vi "PH_PSDBController.set i Attr and open Services.vi"(0 "i ref in":refnum<vi>, 5 "error in":errorcluster) -> (14 "i ref out":refnum<vi>, 16 "i Attributes":T1={"GUI Refs"={"Data Status"=refnum, "Current Shot ID"=refnum, "active Subsystems"=refnum, "Experiment Description"=refnum, "Shot Comment"=refnum, "Experiment"=refnum, "Shottype"=refnum, "Sequencer SM State"=refnum, "Instances with Errors"=refnum}, "Service ID Shot ID"=-1, "Service ID wanted Subsystem"=-1, "Data Status"=0, "Shotinformation"={"Current Experiment ID"=-1, "Current Shot Type"=-1, "Current Comment"=""}, "Data taking?"=FALSE, "Service ID current Shottype"=-1, "Service ID current Experiment"=-1, "Service ID currentShot Comment"=-1, "Service ID possible Shottypes"=-1, "Service ID possible Experiments"=-1, "possible Experiments"=[], "possible Shottypes"=[], "List"=[], "Subsystems Off?"={"PHELIX_Beamline_fs_YLF_BL_Status"=FALSE, "PHELIX_Beamline_ns_BL_Status"=FALSE, "PHELIX_Beamline_PA_Input_BL_Status"=FALSE, "PHELIX_Beamline_PA_MA_BL_Status"=FALSE, "PHELIX_Beamline_MA_Z6_BL_Status"=FALSE, "PHELIX_Beamline_MA_LB_BL_Status"=FALSE, "PHELIX_Beamline_PA_LL_BL_Status"=FALSE}, "PSDB Credentials"={"PW"="N/A", "ID"="N/A", "DS"="N/A"}} {"List"."Info"."Data Status" items=["no info", "no Data collection", "no problem", "Error getting the ID", "Error writing Data", "Error getting the subsystem", "Error getting the Shot ID", "Error getting the Shot Types", "Error getting the Experiments", "Error verifying wanted Shottype", "Error verifying wanted Experiment"]; "Data Status" items=["no info", "no Data collection", "no problem", "Error getting the ID", "Error writing Data", "Error getting the subsystem", "Error getting the Shot ID", "Error getting the Shot Types", "Error getting the Experiments", "Error verifying wanted Shottype", "Error verifying wanted Experiment"]}, 19 "error out":errorcluster)   [LabVIEW 2014, in "PH_PSDBController.lvlib"]
doc: "In this VI own attributes are set."
uses:
  PH_PSDBController.lvlib
  PH_PSDBController.i attribute.ctl
  PH_Basics/PH_PSDBWriter/PH_PSDBWriter.Data Status.ctl
  CSlibraries-extern/psdb_lv/PSDB_Info.ctl
  PH_Basics/PH_Common/Connection/PH_Connection.PSDB Credentials.ctl
  PH_Devices/PH_Beckhoff_Common/PH_Beckhoff_Common.former PSDB classes.ctl
  PH_Basics/PH_Common/PH_Common.lvlib
  PH_Devices/PH_Beckhoff_Common/PH_Beckhoff_Common.lvlib
  PH_Basics/PH_PSDBWriter/PH_PSDBWriter.lvlib
  CSlibraries-extern/psdb_lv/PSDB.lvlib
  CSlibraries/UtilityLib/UtilityLib.lvlib
  CSlibraries-extern/DimLVEvent/LVDimInterface/LVDimInterface.lvlib
  CS_Core/CSSystem/CSSystemLib/CSSystemLib.lvlib
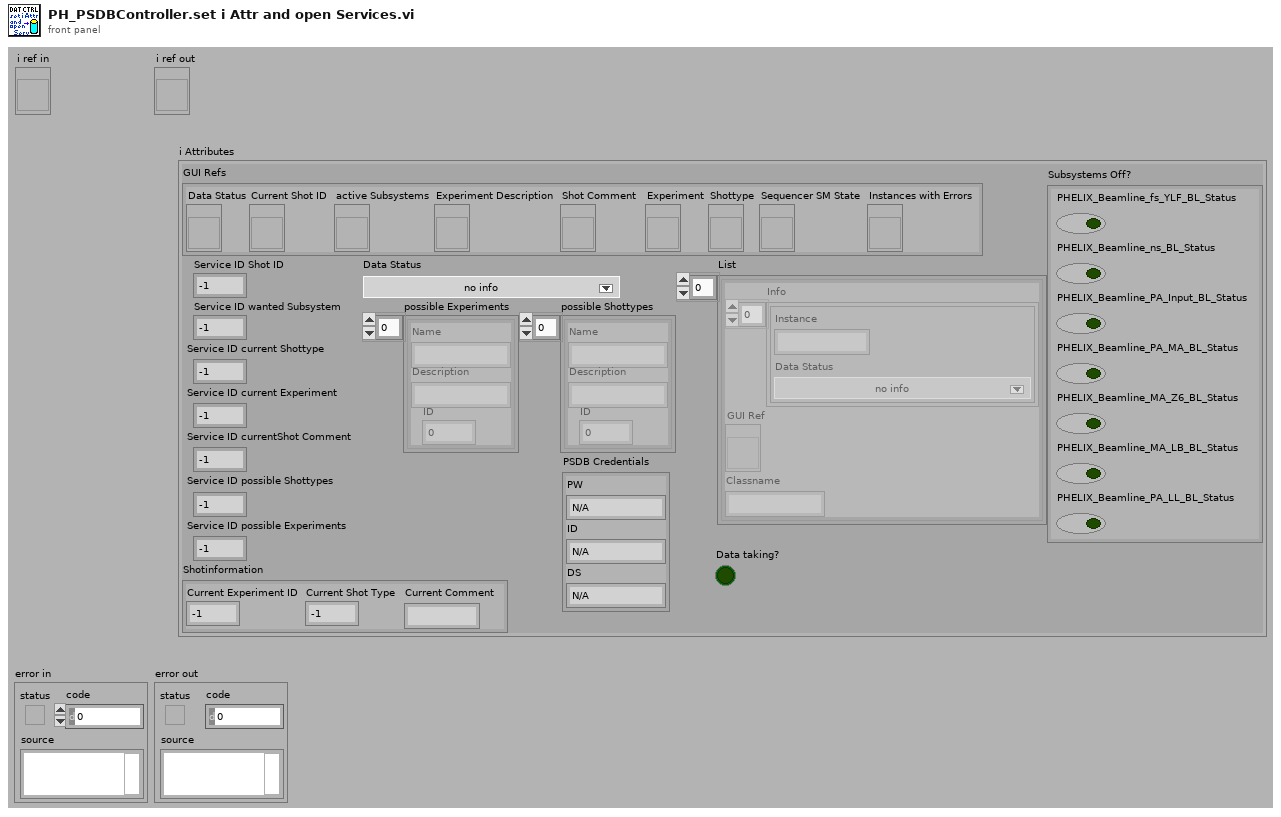
[diagram p1: front panel]
types:
  T1 = typedef "PH_PSDBController.lvlib/PH_PSDBController.i attribute.ctl" = cluster{"GUI Refs":cluster{"Data Status":refnum<vi>, "Current Shot ID":refnum<vi>, "active Subsystems":refnum<vi>, "Experiment Description":refnum<vi>, "Shot Comment":refnum<vi>, "Experiment":refnum<vi>, "Shottype":refnum<vi>, "Sequencer SM State":refnum<vi>, "Instances with Errors":refnum<vi>}, "Service ID Shot ID":i32, "Service ID wanted Subsystem":i32, "Data Status":T2, "Shotinformation":cluster{"Current Experiment ID":i32, "Current Shot Type":i32, "Current Comment":string}, "Data taking?":bool, "Service ID current Shottype":i32, "Service ID current Experiment":i32, "Service ID currentShot Comment":i32, "Service ID possible Shottypes":i32, "Service ID possible Experiments":i32, "possible Experiments":T3[], "possible Shottypes":T3[], "List":cluster{"Info":cluster{"Instance":string, "Data Status":T2}[], "GUI Ref":refnum<vi>, "Classname":string}[], "Subsystems Off?":cluster{"PHELIX_Beamline_fs_YLF_BL_Status":bool, "PHELIX_Beamline_ns_BL_Status":bool, "PHELIX_Beamline_PA_Input_BL_Status":bool, "PHELIX_Beamline_PA_MA_BL_Status":bool, "PHELIX_Beamline_MA_Z6_BL_Status":bool, "PHELIX_Beamline_MA_LB_BL_Status":bool, "PHELIX_Beamline_PA_LL_BL_Status":bool}, "PSDB Credentials":T4}
  T2 = typedef "PH_PSDBWriter.lvlib/PH_PSDBWriter.Data Status.ctl" = i16
  T3 = typedef "PSDB.lvlib/PSDB_Info.ctl" = cluster{"Name":string, "Description":string, "ID":i32}
  T4 = typedef "PH_Common.lvlib/PH_Connection.PSDB Credentials.ctl" = cluster{"PW":string, "ID":string, "DS":string}
  T5 = cluster{"Info":cluster{"Instance":string, "Data Status":T2}[], "GUI Ref":refnum<vi>, "Classname":string}
  T6 = typedef "PH_Beckhoff_Common.lvlib/PH_Beckhoff_Common.former PSDB classes.ctl" = enum16{"PP Conductivity", "PP Mercury", "PA Chiller"}
  T7 = cluster{"Info":cluster{"Instance":string, "Data Status":T2}[], "GUI Ref":refnum<vi>, "Classname":string}[]
  T8 = cluster{"Instancename":string, "Classname":string}
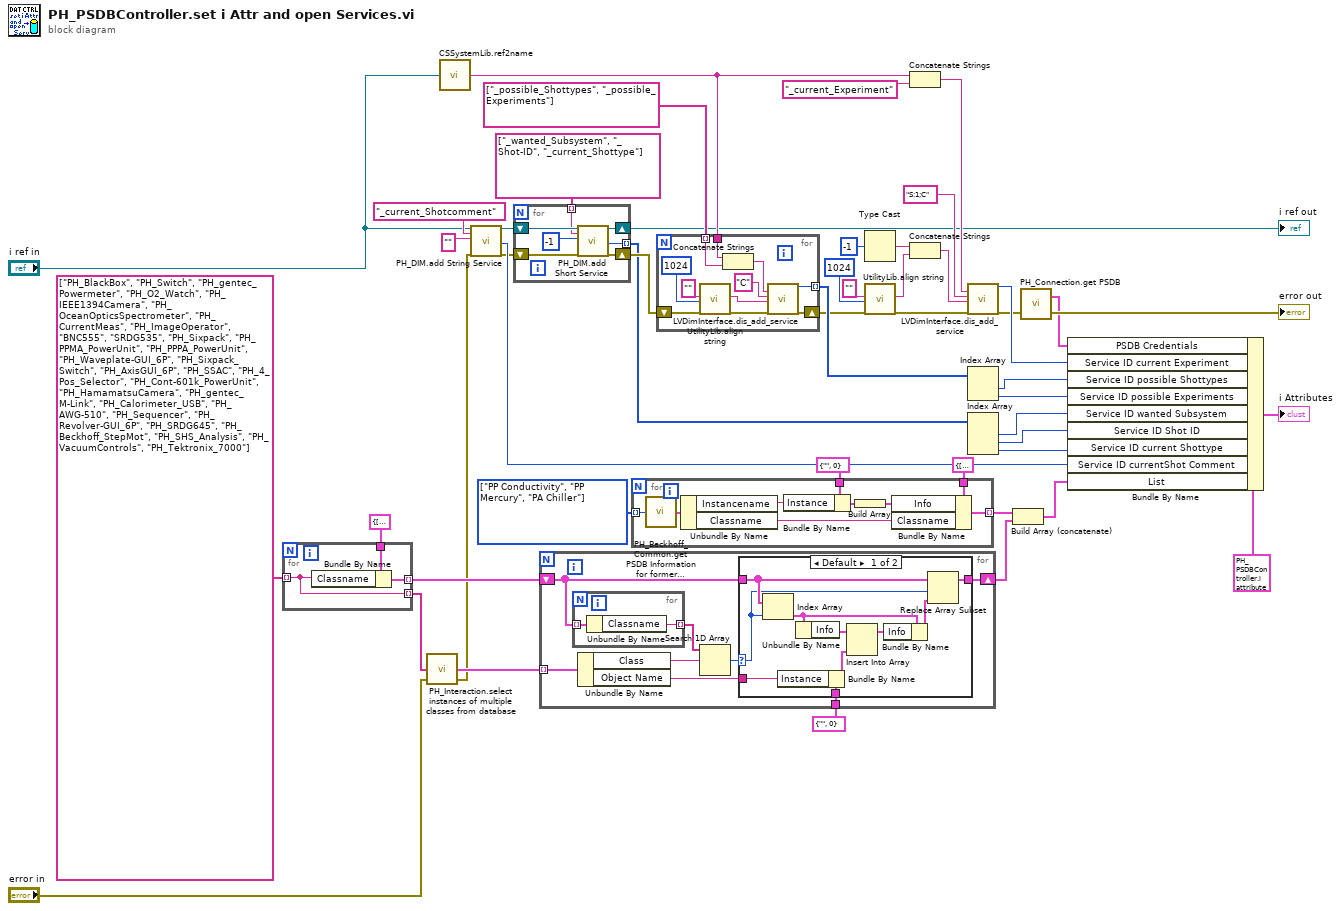
[diagram p0: block diagram]
diagram:
  w45 = T6[] [enum."PP Conductivity", enum."PP Mercury", enum."PA Chiller"] items=["PP Conductivity", "PP Mercury", "PA Chiller"]
  n1 = for {
    tunnel: string[] ["PH_BlackBox", "PH_Switch", "PH_gentec_Powermeter", "PH_O2_Watch", "PH_IEEE1394Camera", "PH_OceanOpticsSpectrometer", "PH_CurrentMeas", "PH_ImageOperator", "BNC555", "SRDG535", "PH_Sixpack", "PH_PPMA_PowerUnit", "PH_PPPA_PowerUnit", "PH_Waveplate-GUI_6P", "PH_Sixpack_Switch", "PH_AxisGUI_6P", "PH_SSAC", "PH_4_Pos_Selector", "PH_Cont-601k_PowerUnit", "PH_HamamatsuCamera", "PH_gentec_M-Link", "PH_Calorimeter_USB", "PH_AWG-510", "PH_Sequencer", "PH_Revolver-GUI_6P", "PH_SRDG645", "PH_Beckhoff_StepMot", "PH_SHS_Analysis", "PH_VacuumControls", "PH_Tektronix_7000"] ("Classes Input") -> [w50] mode=indexing
    tunnel: T5 {"Info"=[], "GUI Ref"=refnum, "Classname"=""} ("Classes") -> [w52]
    tunnel: [w51] -> w46 mode=indexing
    tunnel: [w50] -> w13 mode=indexing
    n2 = Bundle By Name(cluster=w52, "Classname"=w50) -> (w51:T5)
  }
  n3 = call "PH_Interaction.select instances of multiple classes from database.vi"("error in (no error)"="error in", "Classes Input"=w13) -> ("error out"=w8:errorcluster, "Query Result"=w48:cluster{"Object Name":string, "Class":string}[])  [unwired: 2 in]
  n4 = call "CSSystemLib.ref2name.vi"("obj refnum"="i ref in") -> ("name"=w37:string)
  n5 = call "PH_DIM.add String Service.vi"("i ref in"="i ref in", "Service Name"="_current_Shotcomment", "String"="" ("stringIn"), "error in (no error)"=w8) -> ("i ref out"=w19:refnum<vi>, "Service ID"=w21:i32, "error out"=w18:errorcluster)  [unwired: 13 in]
  n6 = for {
    shift-right: [w56] -> w4
    shift-left: w19 -> [w57]
    shift-right: [w58] -> w35
    shift-left: w18 -> [w59]
    tunnel: string[] ["_wanted_Subsystem", "_Shot-ID", "_current_Shottype"] -> [w55] mode=indexing
    tunnel: [w54] -> w15 mode=indexing
    n7 = call "PH_DIM.add Short Service.vi"("i ref in"=w57, "Service Name"=w55, "Number"=i16 -1, "error in (no error)"=w59) -> ("i ref out"=w56:refnum<vi>, "Service ID"=w54:i32, "error out"=w58:errorcluster)  [unwired: 13 in]
  }
  "i ref out" <- w4
  n8 = for {
    tunnel: w48 -> [w67] mode=indexing
    shift-right: [w61] -> w47
    shift-left: w46 -> [w63]
    tunnel: cluster{"Instance":string, "Data Status":T2} {"Instance"="", "Data Status"=0} ("Dummy") -> [w60]
    n9 = for {
      tunnel: w63 -> [w80] mode=indexing
      tunnel: [w79] -> w66 mode=indexing
      n10 = Unbundle By Name(w80) -> ("Classname"=w79:string)
    }
    n11 = Unbundle By Name(w67) -> ("Class"=w65:string, "Object Name"=w62:string)
    n12 = Search 1D Array(1D array=w66, element=w65) -> (index of element=w64:i32)  [unwired: 1 in]
    n13 = case shown="Default" w64 {
      selector: w64 -> [w74 _]
      tunnel: w63 -> [w76 w78]
      tunnel: w62 -> [w77 _]
      tunnel: [w75 w78] -> w61
      tunnel: w60 -> [w68 _]
      frame Default {
        n14 = Index Array(array=w76, index=w74) -> (element=w72:T5)
        n15 = Bundle By Name(cluster=w68, "Instance"=w77) -> (w69:cluster{"Instance":string, "Data Status":T2})
        n16 = Unbundle By Name(w72) -> ("Info"=w71:cluster{"Instance":string, "Data Status":T2}[])
        n17 = Insert Into Array(array=w71, new element=w69) -> (w70:cluster{"Instance":string, "Data Status":T2}[])  [unwired: 1 in]
        n18 = Bundle By Name(cluster=w72, "Info"=w70) -> (w73:T5)
        n19 = Replace Array Subset(array=w76, new element=w73, index=w74) -> (w75:T7)
      }
      frame -1 {
      }
    }
  }
  n20 = for {
    tunnel: w45 -> [w89] mode=indexing
    tunnel: T5 {"Info"=[], "GUI Ref"=refnum, "Classname"=""} ("Classes") -> [w87]
    tunnel: cluster{"Instance":string, "Data Status":T2} {"Instance"="", "Data Status"=0} ("Dummy") -> [w85]
    tunnel: [w81] -> w12 mode=indexing
    n21 = call "PH_Beckhoff_Common.get PSDB Information for former classes.vi"("PSDB Classes"=w89) -> ("PSDB Information"=w88:T8)
    n22 = Unbundle By Name(w88) -> ("Instancename"=w82:string, "Classname"=w86:string)
    n23 = Bundle By Name(cluster=w85, "Instance"=w82) -> (w84:cluster{"Instance":string, "Data Status":T2})
    n24 = Build Array(w84) -> (w83:cluster{"Instance":string, "Data Status":T2}[])
    n25 = Bundle By Name(cluster=w87, "Info"=w83, "Classname"=w86) -> (w81:T5)
  }
  n26 = for {
    shift-right: [w98] -> w36
    shift-left: w35 -> [w99]
    tunnel: w37 -> [w97]
    tunnel: string[] ["_possible_Shottypes", "_possible_Experiments"] -> [w95] mode=indexing
    tunnel: [w90] -> w39 mode=indexing
    n27 = call "UtilityLib.align string.vi"("stringIn"="", "stringLength (80)"=u16 1024, "error in (no error)"=w99) -> ("stringOut"=w93:string, "error out"=w100:errorcluster)  [unwired: 15 in]
    n28 = Concatenate Strings(w97, w95) -> (w96:string)
    n29 = call "LVDimInterface.dis_add_service.vi"("serviceName"=w96, "typeDescriptor"="C", "data"=w93, "error in (no error)"=w100) -> ("my_serviceID"=w90:i32, "error out"=w98:errorcluster)  [unwired: 14 in]
  }
  n30 = Type Cast(x=i16 -1 ("Number")) -> (*(type *) &x=w23:string)  [unwired: 1 in]
  n31 = call "UtilityLib.align string.vi"("stringIn"="", "stringLength (80)"=u16 1024, "error in (no error)"=w36) -> ("stringOut"=w33:string, "error out"=w34:errorcluster)  [unwired: 15 in]
  n32 = Concatenate Strings(w37, "_current_Experiment" ("Service Name")) -> (w28:string)
  n33 = Concatenate Strings(w23, w33) -> (w30:string)
  n34 = call "LVDimInterface.dis_add_service.vi"("serviceName"=w28, "typeDescriptor"="S:1;C" ("Service Name"), "data"=w30, "error in (no error)"=w34) -> ("my_serviceID"=w29:i32, "error out"=w3:errorcluster)  [unwired: 14 in]
  n35 = Index Array(array=w39) -> (element #1=w40:i32, element #2=w41:i32)  [unwired: 2 in]
  n36 = Index Array(array=w15) -> (element #1=w16:i32, element #2=w17:i32, element #3=w22:i32)  [unwired: 3 in]
  n37 = Build Array (concatenate)(w12, w47) -> (w6:T7)
  n38 = call "PH_Connection.get PSDB.vi"("error in (no error)"=w3) -> ("error out"=→"error out":errorcluster, "PSDB Credentials"=w1:T4)  [unwired: 1 in]
  n39 = Bundle By Name(cluster=T1 {"GUI Refs"={"Data Status"=refnum, "Current Shot ID"=refnum, "active Subsystems"=refnum, "Experiment Description"=refnum, "Shot Comment"=refnum, "Experiment"=refnum, "Shottype"=refnum, "Sequencer SM State"=refnum, "Instances with Errors"=refnum}, "Service ID Shot ID"=0, "Service ID wanted Subsystem"=0, "Data Status"=0, "Shotinformation"={"Current Experiment ID"=0, "Current Shot Type"=0, "Current Comment"=""}, "Data taking?"=FALSE, "Service ID current Shottype"=0, "Service ID current Experiment"=0, "Service ID currentShot Comment"=0, "Service ID possible Shottypes"=0, "Service ID possible Experiments"=0, "possible Experiments"=[], "possible Shottypes"=[], "List"=[], "Subsystems Off?"={"PHELIX_Beamline_fs_YLF_BL_Status"=FALSE, "PHELIX_Beamline_ns_BL_Status"=FALSE, "PHELIX_Beamline_PA_Input_BL_Status"=FALSE, "PHELIX_Beamline_PA_MA_BL_Status"=FALSE, "PHELIX_Beamline_MA_Z6_BL_Status"=FALSE, "PHELIX_Beamline_MA_LB_BL_Status"=FALSE, "PHELIX_Beamline_PA_LL_BL_Status"=FALSE}, "PSDB Credentials"={"PW"="N/A", "ID"="N/A", "DS"="N/A"}} ("i Attributes"), "PSDB Credentials"=w1, "Service ID current Experiment"=w29, "Service ID possible Shottypes"=w40, "Service ID possible Experiments"=w41, "Service ID wanted Subsystem"=w16, "Service ID Shot ID"=w17, "Service ID current Shottype"=w22, "Service ID currentShot Comment"=w21, "List"=w6) -> (→"i Attributes":T1)
